vi "MDML_publish_vector_data.vi"(7 "connMeta 6":T1, 8 "error in (no error)":errorcluster, 9 "data":T3, 10 "Device ID":string, 11 "Experiment ID in":string) -> (0 "error out":errorcluster)   [LabVIEW 2018]
uses:
  vector_data.ctl
  Downloads/mqtt_lv2013_201708181938/mqtt_lv2013/mqtt Folder/src/class/mqtt/mqttTypedef/mqttConnectionMeta.ctl
  Downloads/mqtt_lv2013_201708181938/mqtt_lv2013/mqtt Folder/src/class/mqtt/mqttTypedef/mqttQOSlevel.ctl
  data_vector_message.ctl
  Downloads/mqtt_lv2013_201708181938/mqtt_lv2013/mqtt Folder/src/class/mqtt/mqtt.lvclass
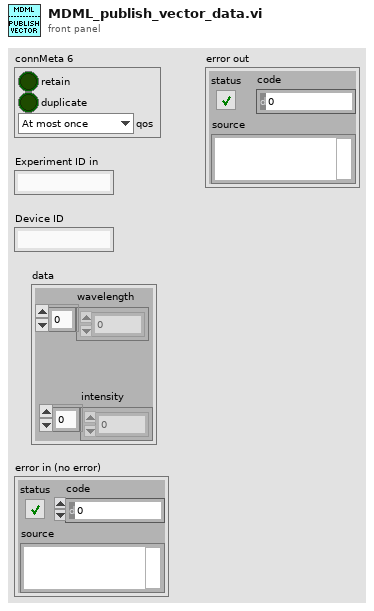
[diagram p1: front panel]
types:
  T1 = typedef "mqttConnectionMeta.ctl" = cluster{"retain":bool, "duplicate":bool, "qos":T2}
  T2 = typedef "mqttQOSlevel.ctl" = enum8{"At most once", "At least once", "Exactly once", "Reserved"}
  T3 = typedef "vector_data.ctl" = cluster{"wavelength":dbl[], "intensity":dbl[]}
  T4 = typedef "data_vector_message.ctl" = cluster{"data_type":string, "influx_measurement":string, "data":cluster{"wavelength":dbl[], "intensity":dbl[]}, "timestamp":string}
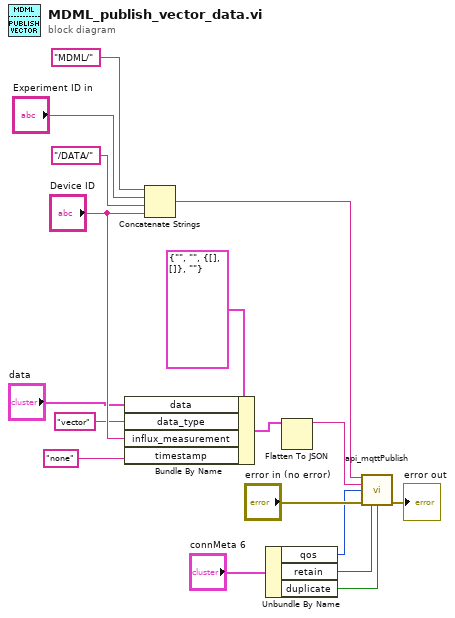
[diagram p0: block diagram]
diagram:
  n1 = Bundle By Name(cluster=T4 {"data_type"="", "influx_measurement"="", "data"={"wavelength"=[], "intensity"=[]}, "timestamp"=""} ("input cluster"), "data"="data", "data_type"="vector", "influx_measurement"="Device ID", "timestamp"="none") -> (w12:T4)
  n2 = Concatenate Strings("MDML/", "Experiment ID in", "/DATA/", "Device ID") -> (w11:string)
  n3 = Unbundle By Name("connMeta 6") -> ("qos"=w7:T2, "retain"=w5:bool, "duplicate"=w6:bool)
  n4 = Flatten To JSON(anything=w12) -> (JSON string=w15:string)  [unwired: 2 in, 1 out]
  n5 = call "api_mqttPublish.vi"("topic"=w11, "value"=w15, "QoS (At most once)"=w7, "error in (no error)"="error in (no error)", "retain(F)"=w5, "duplicate(F)"=w6) -> ("error out"=→"error out":errorcluster)  [unwired: 8 in, 1 out]
